vi "Warehouse-Main.vi"() -> ()   [LabVIEW 2017]
uses:
  Sub VIs/Control/State machine.ctl
  <vilib>/Utility/miscctls.llb/LVPointTypeDef.ctl
  <vilib>/addons/database/Connection.llb/DB Tools Open Connec (Path).vi
  <vilib>/addons/database/Connection.llb/Conn Execute.vi
  <vilib>/addons/database/Recordset.llb/Rec Fetch Recordset Data (R).vi
  <vilib>/addons/database/Recordset.llb/Rec Destroy - Connection.vi
  <vilib>/addons/database/_DB Variant To Data/Database Variant To Data.xnode
  <vilib>/Utility/config.llb/NI_LVConfig.lvlib
  <vilib>/addons/database/NI_Database_API.lvlib
panel:
  out "local":T1
  out "server":T1
  out "warehouse database table":string[](array[string])
  in  "Tab Control":enum32{"Main", "Debug"}(tab)
  out "Network":bool
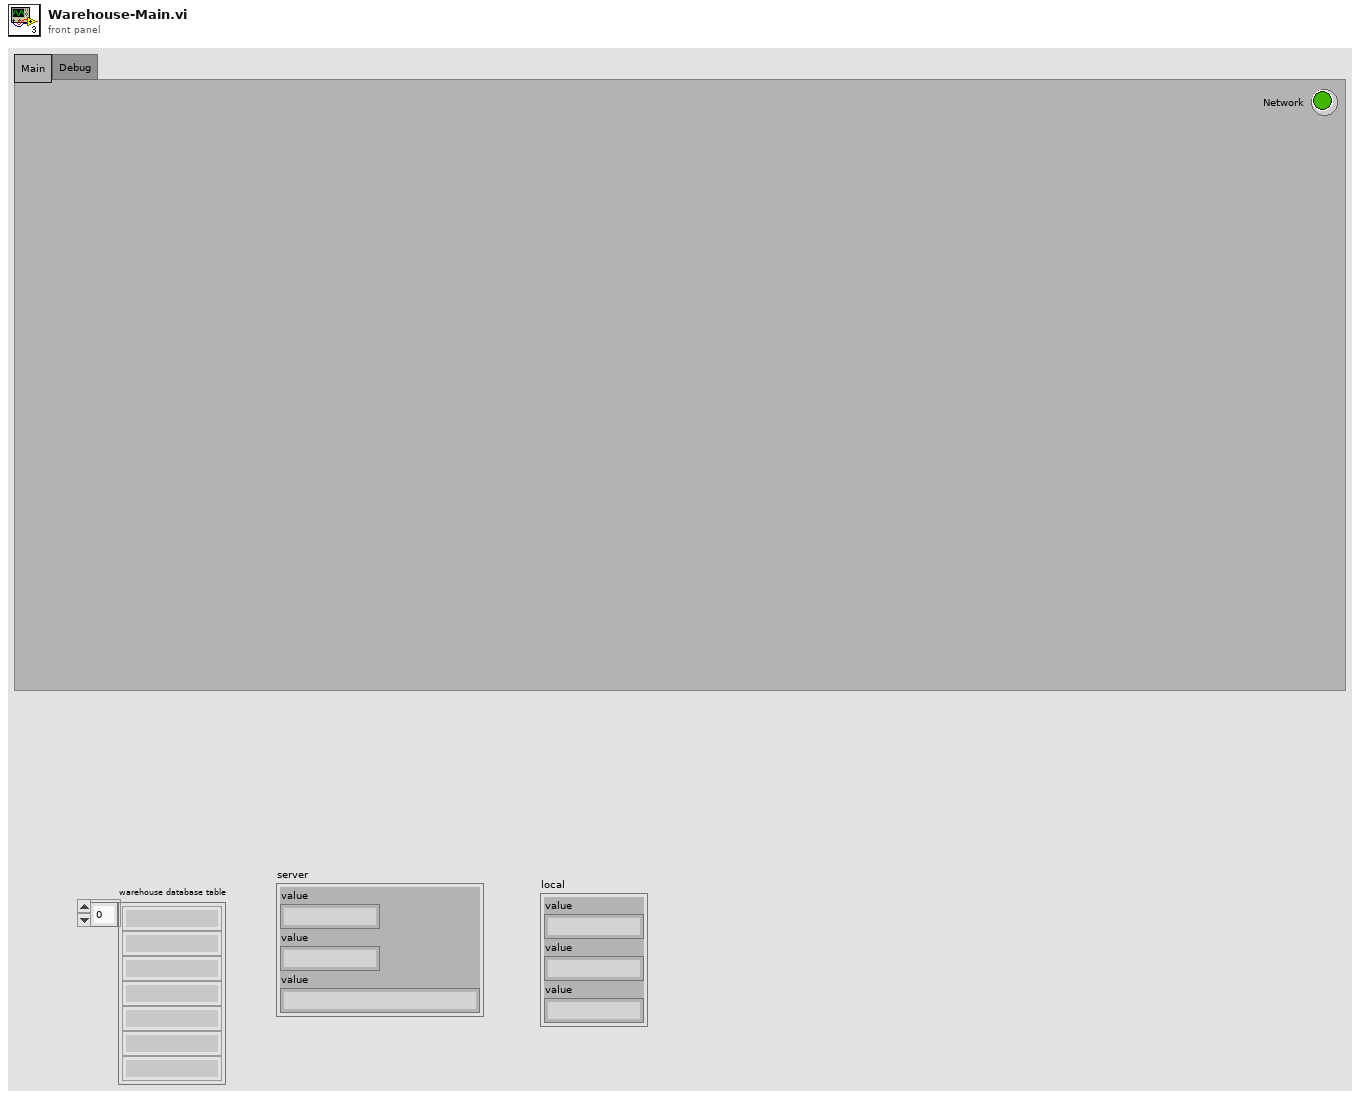
[diagram p1: front panel]
types:
  T1 = cluster{"value":string, "value":string, "value":string}
  T2 = typedef "LVPointTypeDef.ctl" = cluster{"Horizontal":i16, "Vertical":i16}
  T3 = typedef "State machine.ctl" = enum16{"Licence check", "Initial", "Log in", "Creat Config file", "Network setting", "Creat database 1", "Creat database 2", "Creat database 3", "Transfer", "Begin", "Exit"}
  T4 = typedef "NI_LVConfig.lvlib/Config Data RefNum.ctl" = refnum<k1>
  T5 = typedef "NI_Database_API.lvlib/Conn ObjectReference.ctl" = refnum<k1>
  T6 = typedef "NI_Database_API.lvlib/Rec ObjectReference.ctl" = refnum<k1>
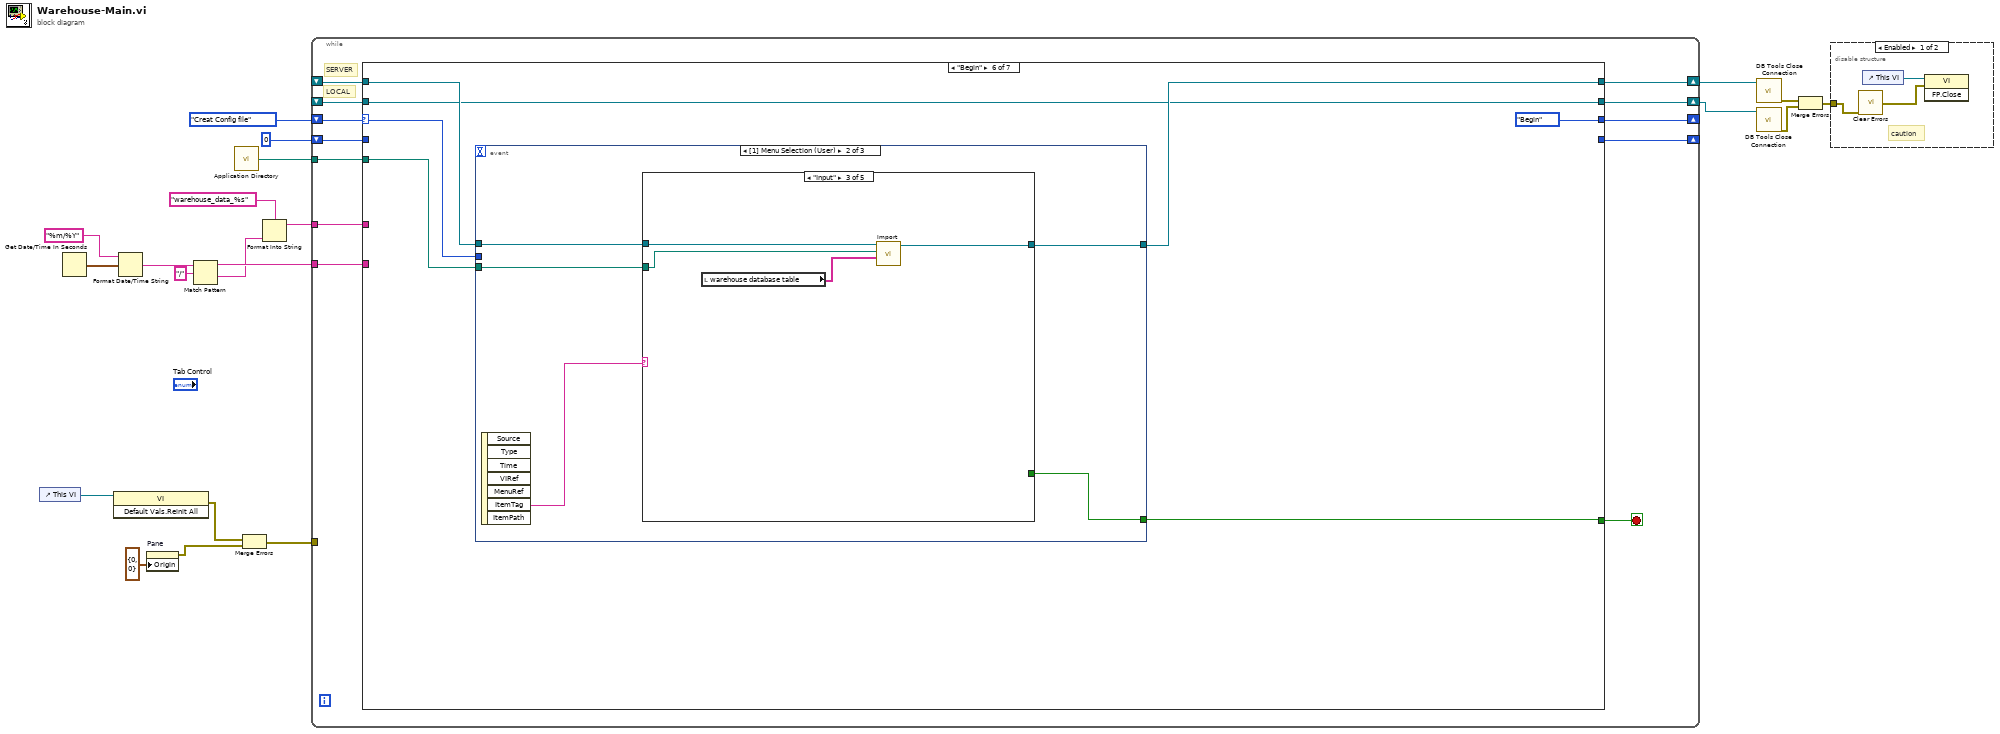
[diagram p0: block diagram]
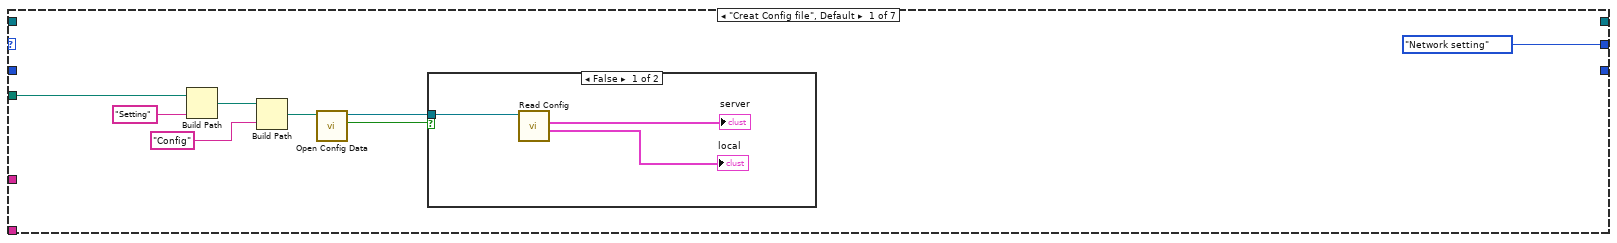
[diagram p3: hidden frame]
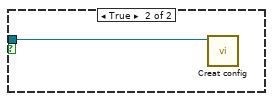
[diagram p4: hidden frame]
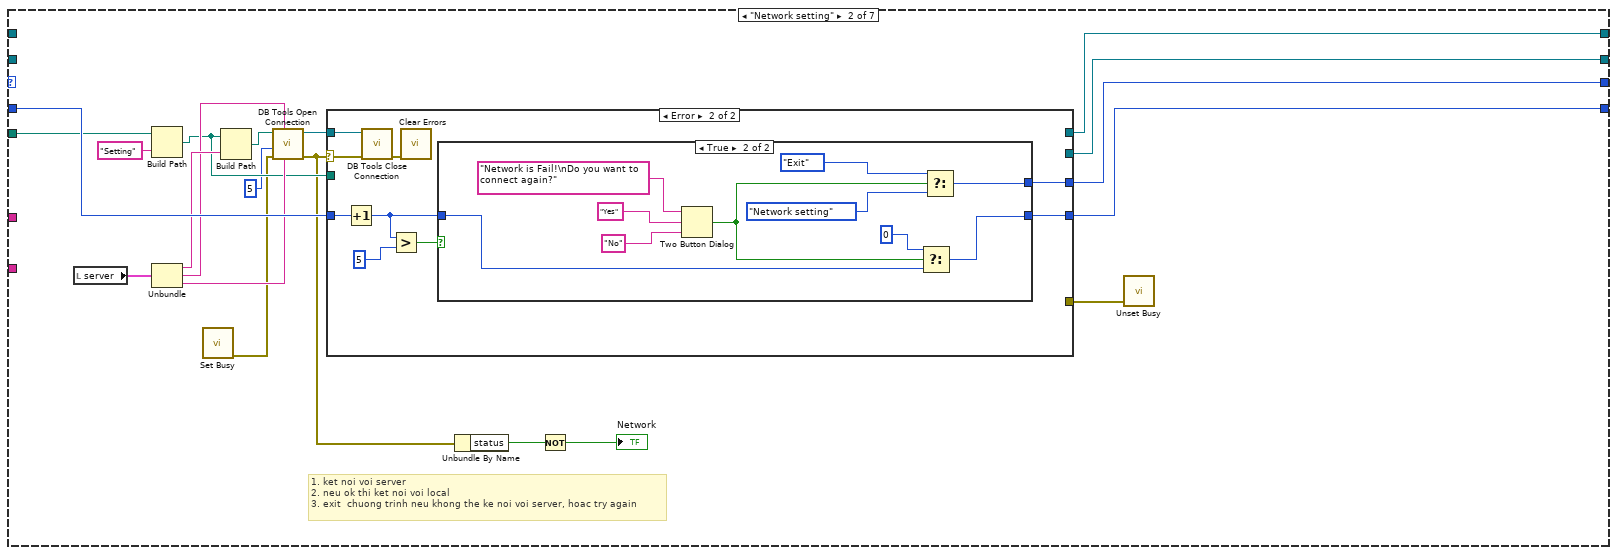
[diagram p5: hidden frame]
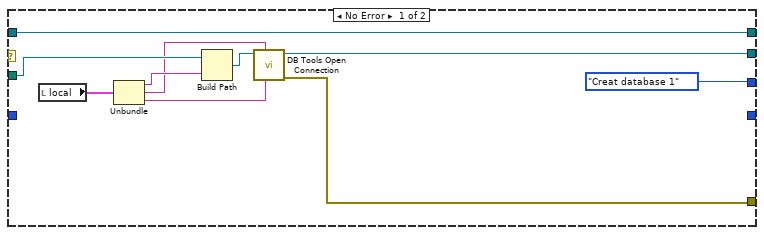
[diagram p6: hidden frame]
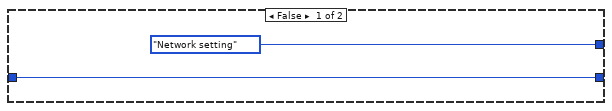
[diagram p7: hidden frame]
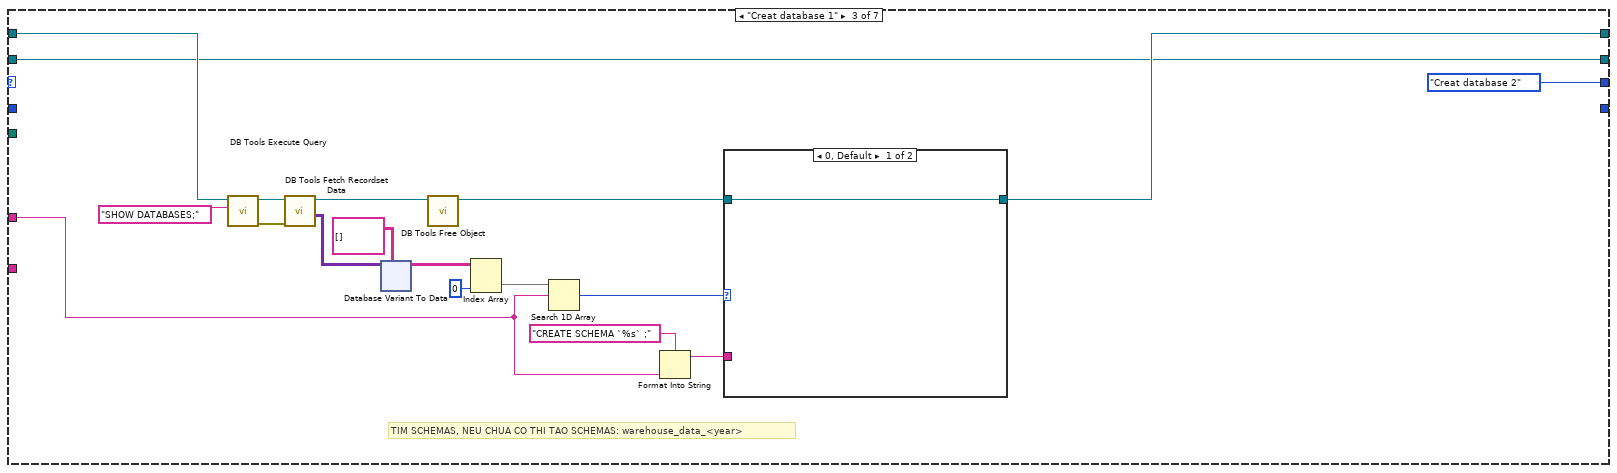
[diagram p8: hidden frame]
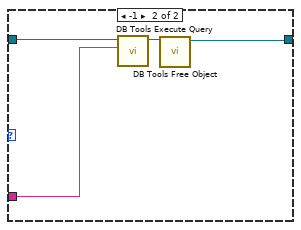
[diagram p9: hidden frame]
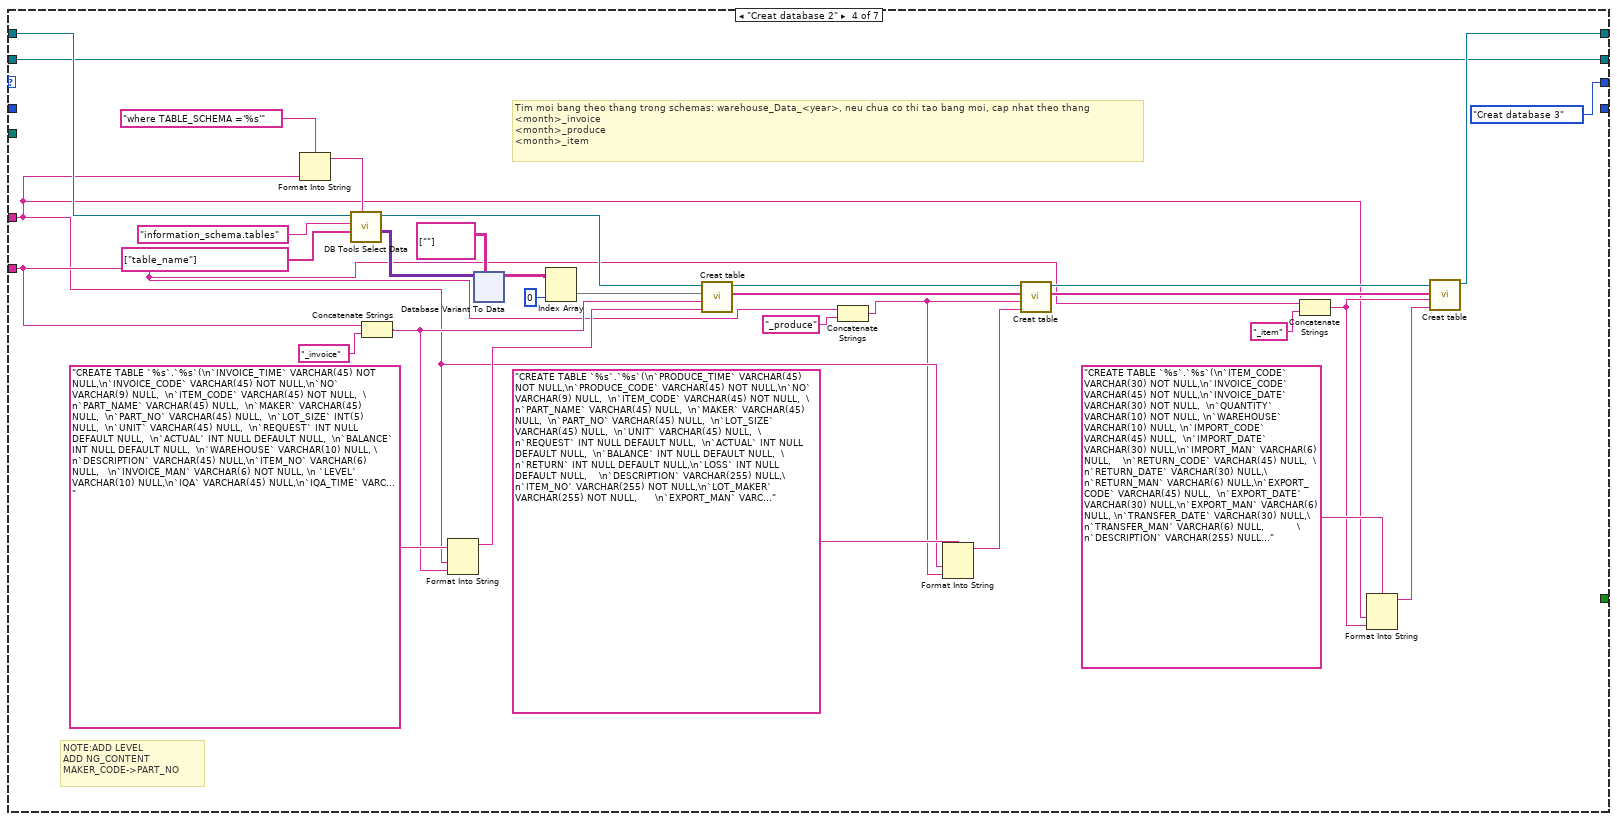
[diagram p10: hidden frame]
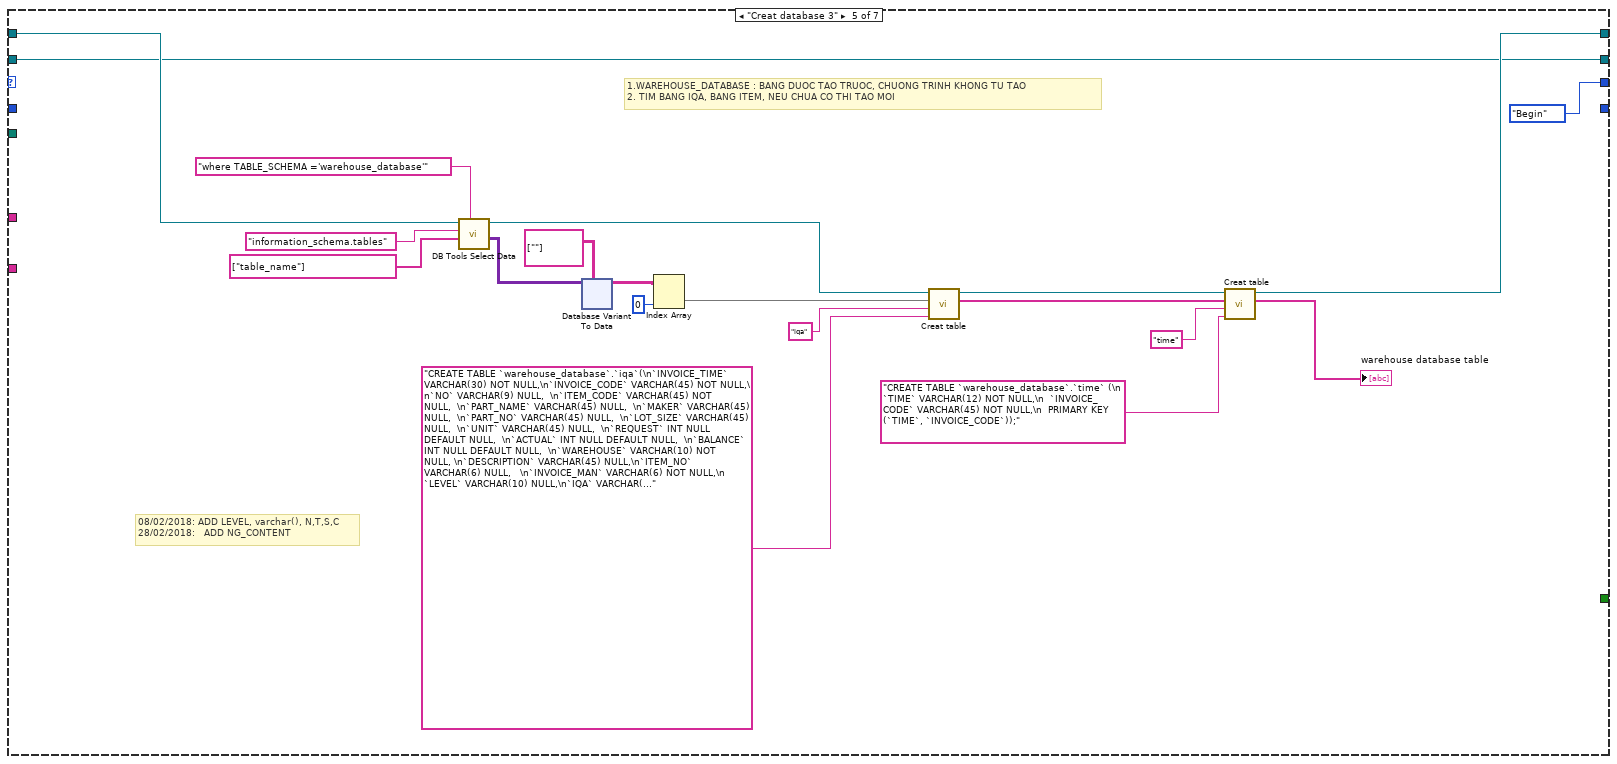
[diagram p11: hidden frame]
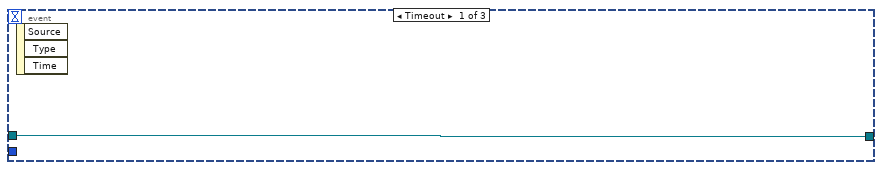
[diagram p12: hidden frame]
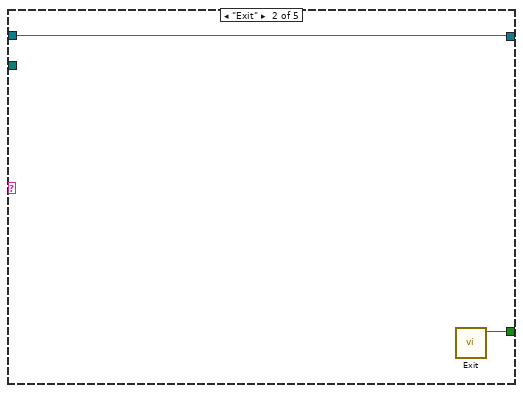
[diagram p14: hidden frame]
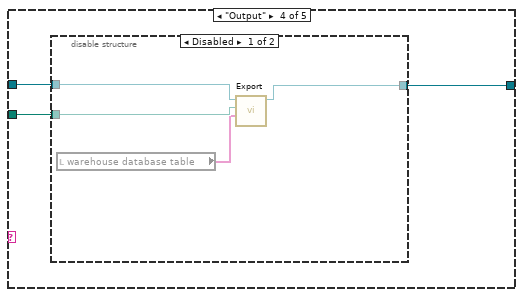
[diagram p15: hidden frame]
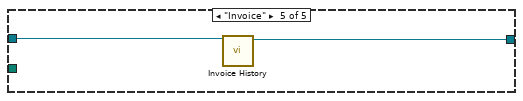
[diagram p17: hidden frame]
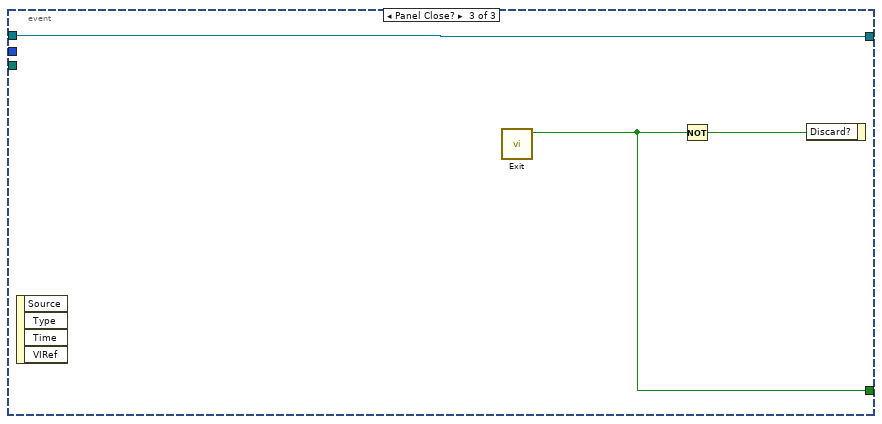
[diagram p18: hidden frame]
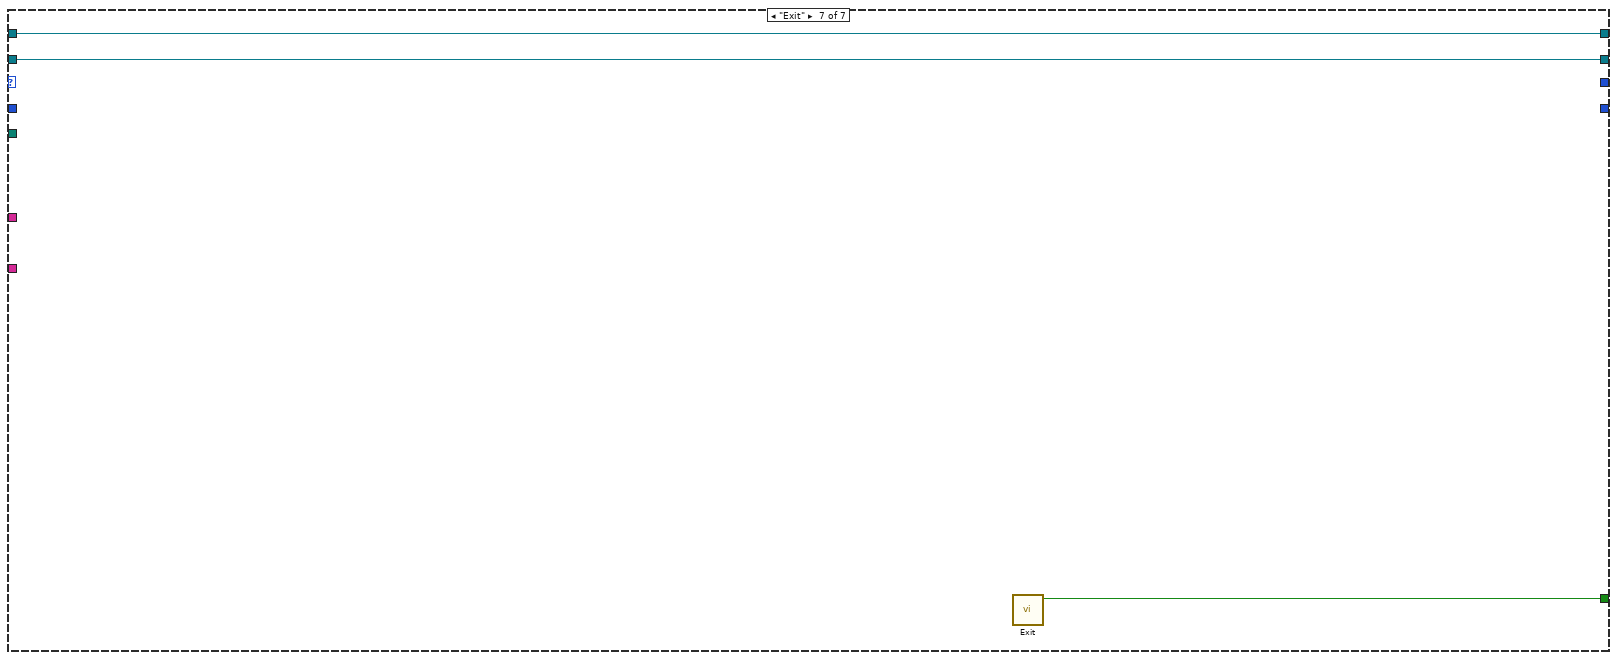
[diagram p19: hidden frame]
diagram:
  n1 = control-ref of="This VI"() -> (w16:refnum<vi>)
  n2 = Get Date/Time In Seconds() -> (seconds since 1Jan1904=w10:timestamp)
  n3 = invoke class="VI" method="Default Vals.Reinit All"(reference=w16) -> (error out=w14:errorcluster)  [unwired: 2 in, 2 out]
  n4 = Format Date/Time String(time format string (%c)="%m/%Y", seconds (now)=w10) -> (date/time string=w9:string)  [unwired: 1 in]
  n5 = property on="Pane" class="Pane"("Origin"=T2 {"Horizontal"=0, "Vertical"=0}) -> (error out=w13:errorcluster)  [unwired: 2 in, 1 out]
  n6 = Match Pattern(string=w9, regular expression="/") -> (before substring=w7:string, after substring=w5:string)  [unwired: 1 in, 2 out]
  n7 = call <vilib>:"Application Directory.vi"() -> ("Application Directory"=w20:path)
  n8 = Merge Errors(w14, w13) -> (w12:errorcluster)
  n9 = Format Into String(format string="warehouse_data_%s", w5) -> (resulting string=w4:string)  [unwired: 2 in, 1 out]
  n10 = while {
    shift-right: [w30] -> _
    shift-left: State_machine."Creat Config file" ("Enum") -> [w32]
    tunnel: w20 -> [w31]
    shift-right: [w29] -> w19
    shift-left: _ -> [w28]
    shift-right: [w26] -> _
    shift-left: 0 -> [w27]
    tunnel: w12 -> [_]
    tunnel: w7 -> [w25]
    tunnel: w4 -> [w24]
    shift-right: [w23] -> w3
    shift-left: _ -> [w22]
    stop <- w33 stop-if-true
    # "LOCAL"
    # "SERVER"
    n11 = case shown="\"Begin\"" w32 {
      selector: w32 -> [_ _ _ _ _ w307 _]
      tunnel: [_ _ _ _ _ w310 w338] -> w33
      tunnel: w31 -> [w40 w60 _ _ _ w305 _]
      tunnel: [State_machine."Network setting" ("Enum") w63 State_machine."Creat database 2" ("Enum") State_machine."Creat database 3" ("Enum") State_machine."Begin" ("Enum") State_machine."Begin" ("Enum") _] -> w30
      tunnel: [_ w64 w104 w178 w257 w308 w337] -> w29
      tunnel: w28 -> [_ _ w109 w195 w244 w309 w337]
      tunnel: w27 -> [_ w62 _ _ _ _ _]
      tunnel: [_ w61 _ _ _ _ _] -> w26
      tunnel: w25 -> [_ _ _ w168 _ _ _]
      tunnel: w24 -> [_ _ w98 w166 _ _ _]
      tunnel: [_ w52 w97 w164 w240 w304 w336] -> w23
      tunnel: w22 -> [_ _ w97 w164 w240 w304 w336]
      frame "Creat Config file", Default {
        n12 = Build Path(base path=w40, name or relative path="Setting") -> (appended path=w38:path)
        n13 = Build Path(base path=w38, name or relative path="Config") -> (appended path=w36:path)
        n14 = call <vilib>:"Open Config Data.vi"("configuration file path"=w36) -> ("file created?"=w35:bool, "refnum"=w34:T4)  [unwired: 8 in, 1 out]
        n15 = case shown="False" w35 {
          tunnel: w34 -> [w44 w45]
          frame False {
            n16 = call "Read Config.vi"("Refnum in"=w44) -> ("local"=→"local":T1, "server"=→"server":T1)  [unwired: 9 in]
          }
          frame True {
            n17 = call "Creat config.vi"("Refnum in"=w45) -> ()  [unwired: 11 in]
          }
        }
      }
      frame "Network setting" {
        # "1. ket noi voi server\n2. neu ok thi ket noi voi local\n3. exit  chuong trinh neu khong the ke noi voi server, hoac try again"
        n18 = local read "server"() -> (w57:T1)
        n19 = Build Path(base path=w60, name or relative path="Setting") -> (appended path=w53:path)
        n20 = Unbundle(w57) -> ("value"=w56:string, "value"=w55:string, "value"=w54:string)
        n21 = call <vilib>:"Set Busy.vi"() -> ("error out"=w47:errorcluster)  [unwired: 10 in, 1 out]
        n22 = Build Path(base path=w53, name or relative path=w56) -> (appended path=w58:path)
        n23 = call-poly <vilib>:"DB Tools Open Connection.vi"("password"=w54, "userID"=w55, "error in (no error)"=w47, "connection timeout (15)"=5, "connection information"=w58) -> ("error out"=w51:errorcluster, "connection reference"=w65:T5)  [unwired: 3 in]
        n24 = case shown="Error" w51 {
          selector: w51 -> [_ w77]
          tunnel: w65 -> [w75 w84]
          tunnel: [w75 _] -> w64
          tunnel: [State_machine."Creat database 1" ("Enum") w80] -> w63
          tunnel: w62 -> [_ w83]
          tunnel: [_ w79] -> w61
          tunnel: w53 -> [w72 _]
          tunnel: [w67 _] -> w52
          tunnel: [w66 _] -> w46
          frame No Error {
            n25 = local read "local"() -> (w71:T1)
            n26 = Unbundle(w71) -> ("value"=w70:string, "value"=w69:string, "value"=w68:string)
            n27 = Build Path(base path=w72, name or relative path=w70) -> (appended path=w73:path)
            n28 = call-poly <vilib>:"DB Tools Open Connection.vi"("password"=w68, "userID"=w69, "connection information"=w73) -> ("error out"=w66:errorcluster, "connection reference"=w67:T5)  [unwired: 5 in]
          }
          frame Error {
            n29 = Increment(x=w83) -> (x+1=w78:i32)
            n30 = call <vilib>:"DB Tools Close Connection.vi"("error in (no error)"=w77, "connection reference"=w84) -> ("error out"=w76:errorcluster)  [unwired: 5 in]
            n31 = Greater?(x=w78, y=5) -> (0:w81:bool)
            n32 = call <vilib>:"Clear Errors.vi"("error in (no error)"=w76) -> ()  [unwired: 5 in, 2 out]
            n33 = case shown="True" w81 {
              tunnel: [State_machine."Network setting" ("Enum") w91] -> w80
              tunnel: [w85 w88] -> w79
              tunnel: w78 -> [w85 w89]
              frame False {
              }
              frame True {
                n34 = Two Button Dialog(message="Network is Fail!\nDo you want to connect again?", 1:"No" ("F button name (\"Cancel\")"), 2:"Yes" ("T button name (\"OK\")")) -> (T button?=w90:bool)
                n35 = Select(t=0, s=w90, f=w89) -> (s? t:f=w88:i32)
                n36 = Select(t=State_machine."Exit" ("Enum"), s=w90, f=State_machine."Network setting" ("Enum")) -> (s? t:f=w91:T3)
              }
            }
          }
        }
        n37 = Unbundle By Name(w51) -> ("status"=w50:bool)
        n38 = Not(x=w50) -> (.not. x?=→"Network":bool)
        n39 = call <vilib>:"Unset Busy.vi"("error in (no error)"=w46) -> ()  [unwired: 10 in, 1 out]
      }
      frame "Creat database 1" {
        # "TIM SCHEMAS, NEU CHUA CO THI TAO SCHEMAS: warehouse_data_<year>"
        n40 = call-poly <vilib>:"DB Tools Execute Query.vi"("SQL query"="SHOW DATABASES;", "connection reference"=w109) -> ("error out"=w114:errorcluster, "recordset reference"=w113:T6)  [unwired: 6 in]
        n41 = call-poly <vilib>:"DB Tools Fetch Recordset Data.vi"("error in (no error)"=w114, "recordset reference"=w113) -> ("recordset data"=w111:variant[][], "recordset reference out"=w112:T6)  [unwired: 3 in, 1 out]
        n42 = xnode "Database Variant To Data"("database variant"=w111, "type"=string[][] []) -> ("data"=w107:string[][])  [unwired: 1 in, 1 out]
        n43 = call-poly <vilib>:"DB Tools Free Object.vi"("recordset reference"=w112) -> ("connection reference"=w105:T5)  [unwired: 9 in, 1 out]
        n44 = Index Array "Index Array"(array=w107, index (col)=0 ("disabled index (col)")) -> (element=w103:string[])  [unwired: 1 in]
        n45 = Search 1D Array(1D array=w103, element=w98) -> (index of element=w102:i32)  [unwired: 1 in]
        n46 = Format Into String(format string="CREATE SCHEMA `%s` ;" ("SQL query"), w98) -> (resulting string=w100:string)  [unwired: 2 in, 1 out]
        n47 = case shown="0, Default" w102 {
          tunnel: w105 -> [w115 w119]
          tunnel: [w115 w118] -> w104
          tunnel: w100 -> [_ w116]
          frame 0, Default {
          }
          frame -1 {
            n48 = call-poly <vilib>:"DB Tools Execute Query.vi"("SQL query"=w116, "connection reference"=w119) -> ("recordset reference"=w117:T6)  [unwired: 6 in, 1 out]
            n49 = call-poly <vilib>:"DB Tools Free Object.vi"("recordset reference"=w117) -> ("connection reference"=w118:T5)  [unwired: 9 in, 1 out]
          }
        }
      }
      frame "Creat database 2" {
        # "NOTE:ADD LEVEL\nADD NG_CONTENT\nMAKER_CODE->PART_NO"
        # "Tim moi bang theo thang trong schemas: warehouse_Data_<year>, neu chua co thi tao bang moi, cap nhat theo thang\n<month>_invoice\n<month>_produce\n<month>_item"
        n50 = Format Into String(format string="where TABLE_SCHEMA ='%s'" ("condition"), w166) -> (resulting string=w173:string)  [unwired: 2 in, 1 out]
        n51 = call <vilib>:"DB Tools Select Data.vi"("condition"=w173, "columns"=string[] ["table_name"], "table"="information_schema.tables", "connection reference"=w195) -> ("data"=w191:variant[][], "connection reference out"=w187:T5)  [unwired: 2 in, 1 out]
        n52 = Concatenate Strings(w168, "_invoice" ("string")) -> (w172:string)
        n53 = Format Into String(format string="CREATE TABLE `%s`.`%s`(\n`INVOICE_TIME` VARCHAR(45) NOT NULL,\n`INVOICE_CODE` VARCHAR(45) NOT NULL,\n`NO` VARCHAR(9) NULL,  \n`ITEM_CODE` VARCHAR(45) NOT NULL,  \n`PART_NAME` VARCHAR(45) NULL,  \n`MAKER` VARCHAR(45) NULL,  \n`PART_NO` VARCHAR(45) NULL,  \n`LOT_SIZE` INT(5) NULL,  \n`UNIT` VARCHAR(45) NULL,  \n`REQUEST` INT NULL DEFAULT NULL,  \n`ACTUAL` INT NULL DEFAULT NULL,  \n`BALANCE` INT NULL DEFAULT NULL,  \n`WAREHOUSE` VARCHAR(10) NULL, \n`DESCRIPTION` VARCHAR(45) NULL,\n`ITEM_NO` VARCHAR(6) NULL,   \n`INVOICE_MAN` VARCHAR(6) NOT NULL, \n `LEVEL` VARCHAR(10) NULL,\n`IQA` VARCHAR(45) NULL,\n`IQA_TIME` VARCHAR(30) NULL,\n`IQA_MAN` VARCHAR(6) NULL,\n`NG_CONTENT` VARCHAR(45) NULL, \nPRIMARY KEY (`INVOICE_TIME`,`INVOICE_CODE`,`ITEM_CODE`))", w166, w172) -> (resulting string=w184:string)  [unwired: 2 in, 1 out]
        n54 = xnode "Database Variant To Data"("database variant"=w191, "type"=string[][] [[""]] ("columns")) -> ("data"=w189:string[][])  [unwired: 1 in, 1 out]
        n55 = Index Array "Index Array"(array=w189, index (col)=0 ("disabled index (col)")) -> (element=w185:string[])  [unwired: 1 in]
        n56 = call "Creat table.vi"("query"=w184, "table name"=w172, "table data"=w185, "Refnum in"=w187) -> ("table data"=w181:string[], "Refnum out"=w183:T5)  [unwired: 6 in]
        n57 = Concatenate Strings(w168, "_produce" ("string")) -> (w165:string)
        n58 = Format Into String(format string="CREATE TABLE `%s`.`%s`(\n`PRODUCE_TIME` VARCHAR(45) NOT NULL,\n`PRODUCE_CODE` VARCHAR(45) NOT NULL,\n`NO` VARCHAR(9) NULL,  \n`ITEM_CODE` VARCHAR(45) NOT NULL,  \n`PART_NAME` VARCHAR(45) NULL,  \n`MAKER` VARCHAR(45) NULL,  \n`PART_NO` VARCHAR(45) NULL,  \n`LOT_SIZE` VARCHAR(45) NULL,  \n`UNIT` VARCHAR(45) NULL,  \n`REQUEST` INT NULL DEFAULT NULL,  \n`ACTUAL` INT NULL DEFAULT NULL,  \n`BALANCE` INT NULL DEFAULT NULL,  \n`RETURN` INT NULL DEFAULT NULL,\n`LOSS` INT NULL DEFAULT NULL,    \n`DESCRIPTION` VARCHAR(255) NULL,\n`ITEM_NO` VARCHAR(255) NOT NULL,\n`LOT_MAKER` VARCHAR(255) NOT NULL,      \n`EXPORT_MAN` VARCHAR(6)  NOT NULL, \n`RETURN_MAN` VARCHAR(6) NOT NULL, \nPRIMARY KEY (`PRODUCE_TIME`,`PRODUCE_CODE`,\n`ITEM_CODE`))", w166, w165) -> (resulting string=w167:string)  [unwired: 2 in, 1 out]
        n59 = call "Creat table.vi"("query"=w167, "table name"=w165, "table data"=w181, "Refnum in"=w183) -> ("table data"=w180:string[], "Refnum out"=w182:T5)  [unwired: 6 in]
        n60 = Concatenate Strings(w168, "_item" ("string")) -> (w171:string)
        n61 = Format Into String(format string="CREATE TABLE `%s`.`%s`(\n`ITEM_CODE` VARCHAR(30) NOT NULL,\n`INVOICE_CODE` VARCHAR(45) NOT NULL,\n`INVOICE_DATE` VARCHAR(30) NOT NULL,  \n`QUANTITY` VARCHAR(10) NOT NULL, \n`WAREHOUSE` VARCHAR(10) NULL, \n`IMPORT_CODE` VARCHAR(45) NULL,  \n`IMPORT_DATE` VARCHAR(30) NULL,\n`IMPORT_MAN` VARCHAR(6) NULL,    \n`RETURN_CODE` VARCHAR(45) NULL,  \n`RETURN_DATE` VARCHAR(30) NULL,\n`RETURN_MAN` VARCHAR(6) NULL,\n`EXPORT_CODE` VARCHAR(45) NULL,  \n`EXPORT_DATE` VARCHAR(30) NULL,\n`EXPORT_MAN` VARCHAR(6) NULL, \n`TRANSFER_DATE` VARCHAR(30) NULL,\n`TRANSFER_MAN` VARCHAR(6) NULL,           \n`DESCRIPTION` VARCHAR(255) NULL,\n`IQA` VARCHAR(5) NULL)", w166, w171) -> (resulting string=w175:string)  [unwired: 2 in, 1 out]
        n62 = call "Creat table.vi"("query"=w175, "table name"=w171, "table data"=w180, "Refnum in"=w182) -> ("Refnum out"=w178:T5)  [unwired: 6 in, 1 out]
      }
      frame "Creat database 3" {
        # "08/02/2018: ADD LEVEL, varchar(), N,T,S,C\n28/02/2018:   ADD NG_CONTENT"
        # "1.WAREHOUSE_DATABASE : BANG DUOC TAO TRUOC, CHUONG TRINH KHONG TU TAO\n2. TIM BANG IQA, BANG ITEM, NEU CHUA CO THI TAO MOI"
        n63 = call <vilib>:"DB Tools Select Data.vi"("condition"="where TABLE_SCHEMA ='warehouse_database'", "columns"=string[] ["table_name"], "table"="information_schema.tables", "connection reference"=w244) -> ("data"=w249:variant[][], "connection reference out"=w243:T5)  [unwired: 2 in, 1 out]
        n64 = xnode "Database Variant To Data"("database variant"=w249, "type"=string[][] [[""]] ("columns")) -> ("data"=w247:string[][])  [unwired: 1 in, 1 out]
        n65 = Index Array(array=w247, index (col)=0 ("disabled index (col)")) -> (element=w242:string[])  [unwired: 1 in]
        n66 = call "Creat table.vi"("query"="CREATE TABLE `warehouse_database`.`iqa`(\n`INVOICE_TIME` VARCHAR(30) NOT NULL,\n`INVOICE_CODE` VARCHAR(45) NOT NULL,\n`NO` VARCHAR(9) NULL,  \n`ITEM_CODE` VARCHAR(45) NOT NULL,  \n`PART_NAME` VARCHAR(45) NULL,  \n`MAKER` VARCHAR(45) NULL,  \n`PART_NO` VARCHAR(45) NULL,  \n`LOT_SIZE` VARCHAR(45) NULL,  \n`UNIT` VARCHAR(45) NULL,  \n`REQUEST` INT NULL DEFAULT NULL,  \n`ACTUAL` INT NULL DEFAULT NULL,  \n`BALANCE` INT NULL DEFAULT NULL,  \n`WAREHOUSE` VARCHAR(10) NOT NULL, \n`DESCRIPTION` VARCHAR(45) NULL,\n`ITEM_NO` VARCHAR(6) NULL,   \n`INVOICE_MAN` VARCHAR(6) NOT NULL,\n `LEVEL` VARCHAR(10) NULL,\n`IQA` VARCHAR(45) NULL,\n`IQA_TIME` VARCHAR(30) NULL,\n`IQA_MAN` VARCHAR(6) NULL, \n`NG_CONTENT`VARCHAR(45) NULL,\nPRIMARY KEY (`INVOICE_TIME`,`INVOICE_CODE`,`ITEM_CODE`))", "table name"="iqa", "table data"=w242, "Refnum in"=w243) -> ("table data"=w255:string[], "Refnum out"=w258:T5)  [unwired: 6 in]
        n67 = call "Creat table.vi"("query"="CREATE TABLE `warehouse_database`.`time` (\n  `TIME` VARCHAR(12) NOT NULL,\n  `INVOICE_CODE` VARCHAR(45) NOT NULL,\n  PRIMARY KEY (`TIME`, `INVOICE_CODE`));", "table name"="time", "table data"=w255, "Refnum in"=w258) -> ("table data"=→"warehouse database table":string[], "Refnum out"=w257:T5)  [unwired: 6 in]
      }
      frame "Begin" {
        n68 = event shown="[1] Menu Selection (User)" {
          selector: _ -> [_ _ _]
          dyn-events: _ -> [_ _ _]
          timeout: _ -> [_ _ _]
          tunnel: [_ w315 w335] -> w310
          tunnel: w309 -> [w311 w314 w333]
          tunnel: [w311 w313 w333] -> w308
          tunnel: w307 -> [_ _ _]
          tunnel: w305 -> [_ w312 _]
          event Timeout {
            n69 = event-data() -> ()  [unwired: 1 in, 3 out]
          }
          event Menu Selection (User) {
            n70 = event-data() -> ("ItemTag"=w316:string)  [unwired: 1 in, 6 out]
            n71 = case shown="\"Input\"" w316 {
              tunnel: [_ w319 _ _ _] -> w315
              tunnel: w314 -> [w317 w318 w323 w326 w332]
              tunnel: [w317 w318 w322 w324 w331] -> w313
              tunnel: w312 -> [_ _ w321 w325 _]
              frame Default {
              }
              frame "Exit" {
                n72 = call "Exit.vi"() -> ("T button?"=w319:bool)  [unwired: 11 in]
              }
              frame "Input" {
                n73 = local read "warehouse database table"() -> (w320:string[])
                n74 = call "Import.vi"("warehosue database table"=w320, "Path"=w321, "connection in"=w323) -> ("connection out"=w322:T5)  [unwired: 8 in]
              }
              frame "Output" {
                n75 = disable-structure shown="Disabled" {
                  disable-tunnel: w326 -> [w330 _]
                  disable-tunnel: w325 -> [w329 _]
                  disable-tunnel: [w328 _] -> w324
                  frame Disabled {
                    n76 = local read "warehouse database table"() -> (w327:string[])
                    n77 = call "Export.vi"("warehosue database table"=w327, "Path"=w329, "connection in"=w330) -> ("connection out"=w328:T5)  [unwired: 8 in]
                  }
                  frame Enabled {
                  }
                }
              }
              frame "Invoice" {
                n78 = call "Invoice History.vi"("reference in"=w332) -> ("reference out"=w331:T5)  [unwired: 10 in]
              }
            }
          }
          event Panel Close? {
            n79 = event-data() -> ()  [unwired: 1 in, 4 out]
            n80 = call "Exit.vi"() -> ("T button?"=w335:bool)  [unwired: 11 in]
            n81 = Not(x=w335) -> (.not. x?=w334:bool)
            n82 = event-data("Discard?"=w334) -> ()  [unwired: 1 in, 1 out]
          }
        }
      }
      frame "Exit" {
        n83 = call "Exit.vi"() -> ("T button?"=w338:bool)  [unwired: 11 in]
      }
    }
  }
  n84 = call <vilib>:"DB Tools Close Connection.vi"("connection reference"=w19) -> ("error out"=w17:errorcluster)  [unwired: 6 in]
  n85 = call <vilib>:"DB Tools Close Connection.vi"("connection reference"=w3) -> ("error out"=w2:errorcluster)  [unwired: 6 in]
  n86 = Merge Errors(w17, w2) -> (w1:errorcluster)
  n87 = disable-structure shown="Enabled" {
    disable-tunnel: w1 -> [w339 _]
    frame Enabled {
      # "caution"
      n88 = call <vilib>:"Clear Errors.vi"("error in (no error)"=w339) -> ("error out"=w340:errorcluster)  [unwired: 5 in, 1 out]
      n89 = control-ref of="This VI"() -> (w341:refnum<vi>)
      n90 = invoke class="VI" method="FP.Close"(reference=w341, error in=w340) -> ()  [unwired: 1 in, 3 out]
    }
    frame Disabled {
    }
  }
